vi "XW UV from U1U2 Psi_eff STD PN.vi"(0 "U1cal (m/s)":dbl[](array[numeric]), 5 "U2cal (m/s)":dbl[](array[numeric])) -> (3 "U (m/s)":dbl[](array[numeric]), 4 "V (m/s)":dbl[](array[numeric]), 6 "Psi1 (deg)":dbl[](array[numeric]), 8 "Psi2 (deg)":dbl[](array[numeric]), 14 "Unconverged points (fraction)":dbl)   [LabVIEW 2010]
uses:
  <vilib>/gmath/NI_Gmath.lvlib
panel:
  out "Checks":dbl[][](graph)
  out "Iters":i32
  in  "maxIter":i32=150
  in  "tol":dbl=1e-06
  # "THIS GRAPH MUST BE RE-ENABLED FROM THE BLOCK DIAGRAM IF NEEDED"
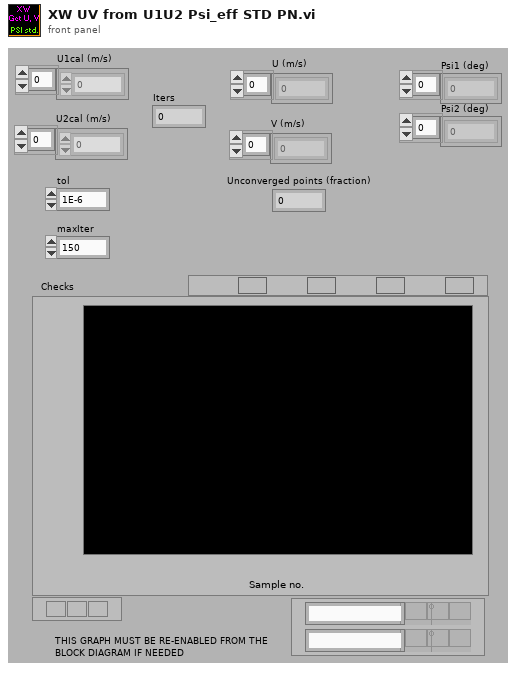
[diagram p1: front panel]
types:
  T1 = typedef "NI_Gmath.lvlib/in_piecewise interp poly control.ctl" = cluster{"x locations":dbl[], "coefficients":dbl[][]}
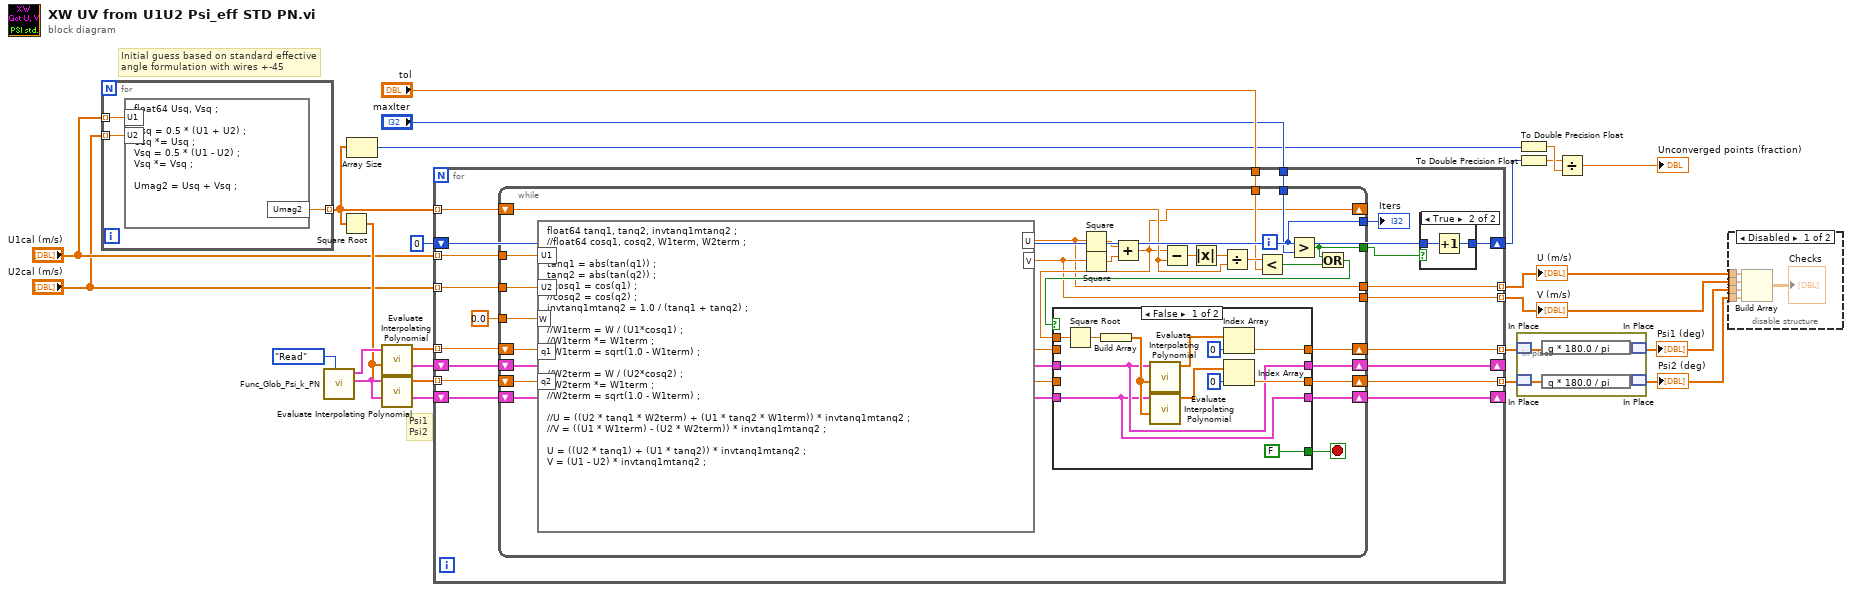
[diagram p0: block diagram]
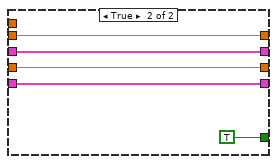
[diagram p4: hidden frame]
diagram:
  # "Initial guess based on standard effective angle formulation with wires +-45"
  # "Psi1\nPsi2"
  n1 = for {
    tunnel: "U1cal (m/s)" -> [w26] mode=indexing
    tunnel: "U2cal (m/s)" -> [w25] mode=indexing
    tunnel: [w24] -> w11 mode=indexing
    n2 = formula code="float64 Usq, Vsq ;\n\nUsq = 0.5 * (U1 + U2) ;\nUsq *= Usq ;\nVsq = 0.5 * (U1 - U2) ;\nVsq *= Vsq ;\n\nUmag2 = Usq + Vsq ;"("U1"=w26, "U2"=w25) -> ("Umag2"=w24:dbl)
  }
  n3 = call "Func_Glob_Psi_k_PN.vi"("Action"=enum16{"Read", "Write"}."Read") -> ("Psi2 coeffs OUT"=w21:T1, "Psi1 coeffs OUT"=w22:T1)  [unwired: 4 in, 2 out]
  n4 = Square Root(x=w11) -> (sqrt(x)=w16:dbl[])
  n5 = Array Size(array=w11) -> (size(s)=w10:i32)
  n6 = call <vilib>:"Evaluate Interpolating Polynomial.vi"("xi"=w16, "piecewise polynomial"=w22) -> ("yi"=w20:dbl[])  [unwired: 9 out]
  n7 = call <vilib>:"Evaluate Interpolating Polynomial.vi"("xi"=w16, "piecewise polynomial"=w21) -> ("yi"=w19:dbl[])  [unwired: 9 out]
  n8 = for {
    tunnel: "U1cal (m/s)" -> [w34] mode=indexing
    tunnel: "U2cal (m/s)" -> [w33] mode=indexing
    shift-right: [w42] -> _
    shift-left: w22 -> [w44]
    shift-right: [w41] -> _
    shift-left: w21 -> [w43]
    tunnel: w20 -> [w46] mode=indexing
    tunnel: w19 -> [w45] mode=indexing
    tunnel: [w40] -> w2 mode=indexing
    tunnel: [w39] -> w5 mode=indexing
    tunnel: "tol" -> [w38]
    tunnel: "maxIter" -> [w37]
    shift-right: [w27] -> w8
    shift-left: 0 -> [w28]
    tunnel: [w32] -> w14 mode=indexing
    tunnel: [w31] -> w15 mode=indexing
    tunnel: w11 -> [w30] mode=indexing
    n9 = while {
      tunnel: w34 -> [w76]
      tunnel: w33 -> [w75]
      shift-right: [w59] -> w32
      shift-left: w46 -> [w57]
      shift-right: [w58] -> w31
      shift-left: w45 -> [w56]
      shift-right: [w61] -> w42
      shift-left: w44 -> [w62]
      shift-right: [w60] -> w41
      shift-left: w43 -> [w63]
      tunnel: [w53] -> w40
      tunnel: [w54] -> w39
      shift-right: [w55] -> _
      shift-left: w30 -> [w70]
      tunnel: w38 -> [w68]
      tunnel: w37 -> [w67]
      tunnel: 0.0 -> [w52]
      tunnel: [w51] -> w35
      tunnel: [w50] -> w29
      i -> [w51]
      stop <- w64 stop-if-true
      n10 = formula code="float64 tanq1, tanq2, invtanq1mtanq2 ;\n//float64 cosq1, cosq2, W1term, W2term ;\n\ntanq1 = abs(tan(q1)) ;\ntanq2 = abs(tan(q2)) ;\n//cosq1 = cos(q1) ;\n//cosq2 = cos(q2) ;\ninvtanq1mtanq2 = 1.0 / (tanq1 + tanq2) ;\n\n//W1term = W / (U1*cosq1) ;\n//W1term *= W1term ;\n//W1term = sqrt(1.0 - W1term) ;\n\n//W2term = W / (U2*cosq2) ;\n//W2term *= W1term ;\n//W2term = sqrt(1.0 - W1term) ;\n\n//U = ((U2 * tanq1 * W2term) + (U1 * tanq2 * W1term)) * invtanq1mtanq2 ;\n//V = ((U1 * W1term) - (U2 * W2term)) * invtanq1mtanq2 ;\n\nU = ((U2 * tanq1) + (U1 * tanq2)) * invtanq1mtanq2 ;\nV = (U1 - U2) * invtanq1mtanq2 ;"("U1"=w76, "U2"=w75, "q1"=w57, "q2"=w56, "W"=w52) -> ("U"=w53:dbl, "V"=w54:dbl)
      n11 = Square(x=w53) -> (x^2=w74:dbl)
      n12 = Square(x=w54) -> (x^2=w73:dbl)
      n13 = Add(x=w74, y=w73) -> (x+y=w55:dbl)
      n14 = Subtract(x=w55, y=w70) -> (x-y=w72:dbl)
      n15 = Absolute Value(x=w72) -> (abs(x)=w71:dbl)
      n16 = Divide(x=w71, y=w70) -> (x/y=w69:dbl)
      n17 = Less?(x=w69, y=w68) -> (x < y?=w66:bool)
      n18 = Greater?(x=w51, y=w67) -> (0:w50:bool)
      n19 = Or(x=w50, y=w66) -> (x .or. y?=w65:bool)
      n20 = case shown="False" w65 {
        tunnel: w55 -> [w87 _]
        tunnel: [FALSE TRUE] -> w64
        tunnel: w63 -> [w77 w91]
        tunnel: w62 -> [w78 w92]
        tunnel: [w78 w92] -> w61
        tunnel: [w77 w91] -> w60
        tunnel: [w83 w90] -> w59
        tunnel: [w79 w89] -> w58
        tunnel: w57 -> [_ w90]
        tunnel: w56 -> [_ w89]
        frame False {
          n21 = Square Root(x=w87) -> (sqrt(x)=w86:dbl)
          n22 = Build Array(w86) -> (w85:dbl[])
          n23 = call <vilib>:"Evaluate Interpolating Polynomial.vi"("xi"=w85, "piecewise polynomial"=w78) -> ("yi"=w82:dbl[])  [unwired: 9 out]
          n24 = call <vilib>:"Evaluate Interpolating Polynomial.vi"("xi"=w85, "piecewise polynomial"=w77) -> ("yi"=w80:dbl[])  [unwired: 9 out]
          n25 = Index Array(array=w82, index=0) -> (element=w83:dbl)
          n26 = Index Array(array=w80, index=0) -> (element=w79:dbl)
        }
        frame True {
        }
      }
    }
    "Iters" <- w35
    n27 = case shown="True" w29 {
      tunnel: w28 -> [w47 w49]
      tunnel: [w47 w48] -> w27
      frame False {
      }
      frame True {
        n28 = Increment(x=w49) -> (x+1=w48:i32)
      }
    }
  }
  "U (m/s)" <- w2
  "V (m/s)" <- w5
  n29 = in-place {
    n30 = in-place-match #1(w14) -> (w95:dbl[])
    n31 = in-place-match #2(w15) -> (w97:dbl[])
    n32 = expression code="q * 180.0 / pi"(w95) -> (w94:dbl[])
    n33 = expression code="q * 180.0 / pi"(w97) -> (w96:dbl[])
    n34 = in-place-match #1(w94) -> (w4:dbl[])
    n35 = in-place-match #2(w96) -> (w3:dbl[])
  }
  "Psi1 (deg)" <- w4
  "Psi2 (deg)" <- w3
  n36 = To Double Precision Float(number=w10) -> (double precision float=w7:dbl)
  n37 = To Double Precision Float(number=w8) -> (double precision float=w6:dbl)
  n38 = Divide(x=w6, y=w7) -> (x/y=→"Unconverged points (fraction)":dbl)
  n39 = disable-structure shown="Disabled" {
    disable-tunnel: w5 -> [w102 _]
    disable-tunnel: w4 -> [w101 _]
    disable-tunnel: w3 -> [w100 _]
    disable-tunnel: w2 -> [w98 _]
    frame Disabled {
      n40 = Build Array(w98, w102, w101, w100) -> (→"Checks":dbl[][])
    }
    frame Enabled {
    }
  }
